vi "CTRE_Phoenix_MotorControl_ConfigReverseLimitSwitch_Enhanced.vi"(0 "CTRE Motor Controller Device Ref":T3={"DeviceStatus"={"status"=FALSE, "code"=0, "source"=""}, "Type"=enum."PWM", "PWM"={"PWM Channel"=enum."PWM 1", "DeadBand"={"Name"="", "maxPositivePwm"=0, "minPositivePwm"=0, "centerPwm"=0, "maxNegativePwm"=0, "minNegativePwm"=0, "angularRange"=0}}, "CAN"={"Device Number"=0, "SetOutput VI Ref"=variant(enum8{"Percent VBus", "Current", "Speed", "Position", "Voltage"} enum."Percent VBus"), "GetOutput VI Ref"=variant(refnum<k1> refnum), "Enable VI Ref"=variant(dbl 12.0), "Disable VI Ref"=variant(enum8{"Percent VBus", "Speed", "Position", "Slave", "Unchanged / Invalid", "Voltage Compensation", "Current", "Motion Profile"} enum."Percent VBus"), "Data"=variant}, "Invert"=FALSE}, 5 "Limit Switch Source":T2, 7 "NormallyOpenOrClosed":T1, 9 "deviceID":i32, 11 "error in (no error)":errorcluster) -> (4 "CTRE Motor Controller Device Ref":T3={"DeviceStatus"={"status"=FALSE, "code"=0, "source"=""}, "Type"=enum."PWM", "PWM"={"PWM Channel"=enum."PWM 1", "DeadBand"={"Name"="", "maxPositivePwm"=0, "minPositivePwm"=0, "centerPwm"=0, "maxNegativePwm"=0, "minNegativePwm"=0, "angularRange"=0}}, "CAN"={"Device Number"=0, "SetOutput VI Ref"=variant(enum8{"Percent VBus", "Current", "Speed", "Position", "Voltage"} enum."Percent VBus"), "GetOutput VI Ref"=variant(refnum<k1> refnum), "Enable VI Ref"=variant(dbl 12.0), "Disable VI Ref"=variant(enum8{"Percent VBus", "Speed", "Position", "Slave", "Unchanged / Invalid", "Voltage Compensation", "Current", "Motion Profile"} enum."Percent VBus"), "Data"=variant}, "Invert"=FALSE}, 15 "error out":errorcluster)   [LabVIEW 2016]
doc: "Configures the reverse limit switch.\n\n<B>Limit Switch Source</B> indicates the source of the limit switch, whether local (feedback connector) or from a remote device.\n\n<B>deviceID</B> must be set if using a remote limit switch."
uses:
  <vilib>/Rock Robotics/WPI/MotorControl/WPI_MotorControlDeviceRef.ctl
  <vilib>/Rock Robotics/WPI/MotorControl/WPI_MotorControlType.ctl
  <vilib>/Rock Robotics/SystemInterfaces/DIO/FPGA_DIOPWMChannel.ctl
  <vilib>/Rock Robotics/WPI/PWM/WPI_PWMDeadband.ctl
  Controls/CTRE_Phoenix_MotorControl_LimitSwitchSource_Local.ctl
  Controls/CTRE_Phoenix_MotorControl_LimitSwitchNormal.ctl
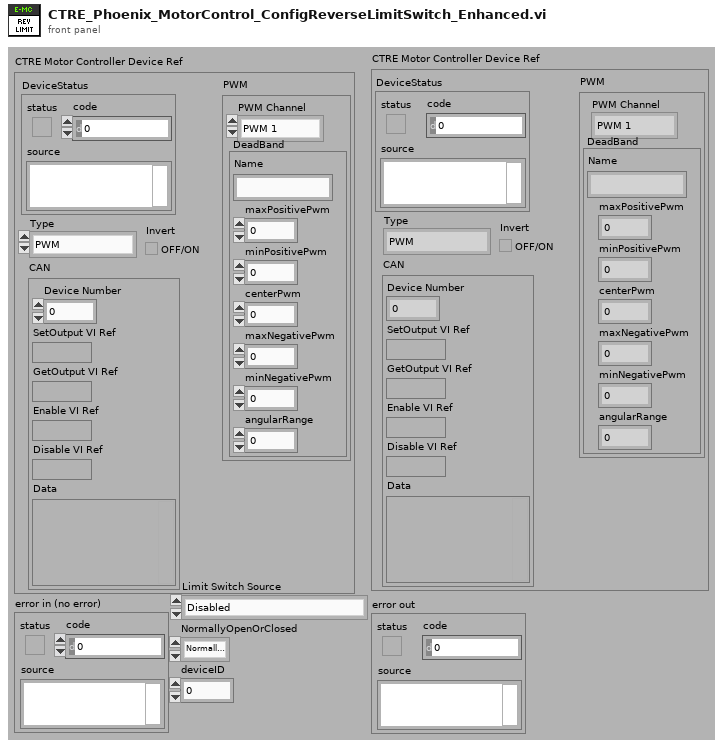
[diagram p1: front panel]
types:
  T1 = typedef "CTRE_Phoenix_MotorControl_LimitSwitchNormal.ctl" = enum16{"Normally Open", "Normally Closed"}
  T2 = typedef "CTRE_Phoenix_MotorControl_LimitSwitchSource_Local.ctl" = enum16{"Disabled", "FeedbackConnector", "RemoteTalonSRX", "RemoteCANifier"}
  T3 = typedef "WPI_MotorControlDeviceRef.ctl" = cluster{"DeviceStatus":errorcluster, "Type":T4, "PWM":cluster{"PWM Channel":T5, "DeadBand":T6}, "CAN":cluster{"Device Number":u8, "SetOutput VI Ref":variant, "GetOutput VI Ref":variant, "Enable VI Ref":variant, "Disable VI Ref":variant, "Data":variant}, "Invert":bool}
  T4 = typedef "WPI_MotorControlType.ctl" = enum16{"PWM", "CAN"}
  T5 = typedef "FPGA_DIOPWMChannel.ctl" = enum8{"PWM 0", "PWM 1", "PWM 2", "PWM 3", "PWM 4", "PWM 5", "PWM 6", "PWM 7", "PWM 8", "PWM 9", "PWM MXP 0", "PWM MXP 1", "PWM MXP 2", "PWM MXP 3", "PWM MXP 4", "PWM MXP 5", "PWM MXP 6", "PWM MXP 7", "PWM MXP 8", "PWM MXP 9", "Invalid"}
  T6 = typedef "WPI_PWMDeadband.ctl" = cluster{"Name":string, "maxPositivePwm":i32, "minPositivePwm":i32, "centerPwm":i32, "maxNegativePwm":i32, "minNegativePwm":i32, "angularRange":u16}
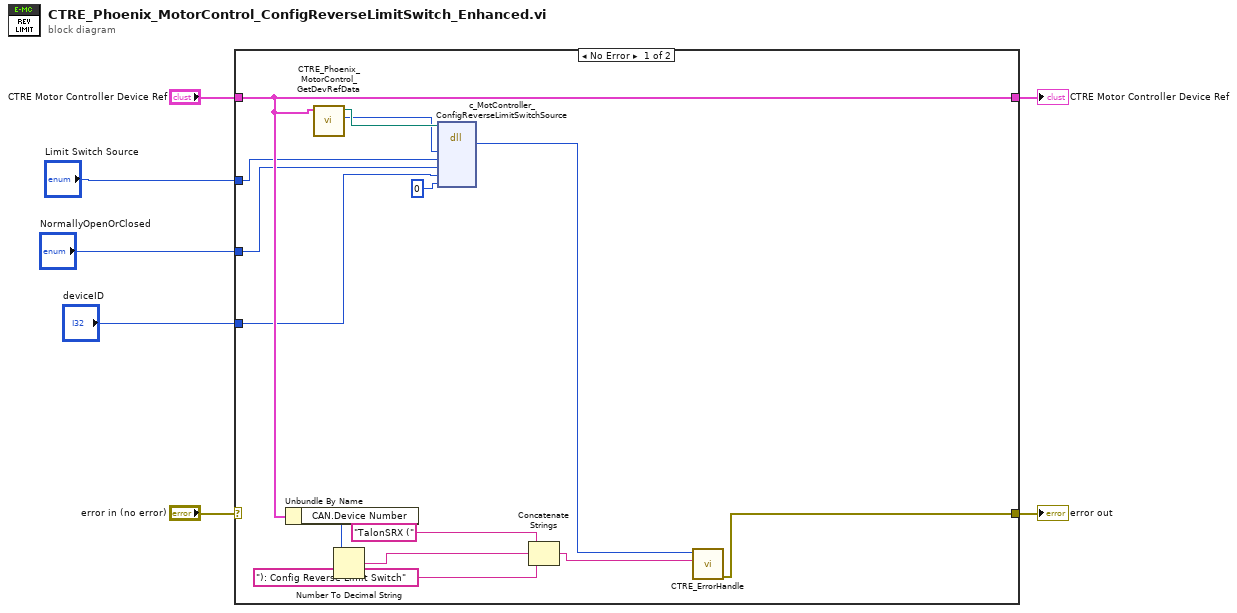
[diagram p0: block diagram]
diagram:
  n1 = case shown="No Error" "error in (no error)" {
    selector: "error in (no error)" -> [_ w23]
    tunnel: [w14 w23] -> w7
    tunnel: "CTRE Motor Controller Device Ref" -> [w17 w22]
    tunnel: [w17 w22] -> w5
    tunnel: "Limit Switch Source" -> [w10 _]
    tunnel: "NormallyOpenOrClosed" -> [w9 _]
    tunnel: "deviceID" -> [w8 _]
    frame No Error {
      n2 = Unbundle By Name(w17) -> ("CAN.Device Number"=w18:u8)
      n3 = call "CTRE_Phoenix_MotorControl_GetDevRefData.vi"("MotorControlDevRef"=w17) -> ("handle"=w11:u64, "Library"=w12:path)  [unwired: 4 in, 5 out]
      n4 = Number To Decimal String(number=w18) -> (decimal integer string=w20:string)  [unwired: 1 in]
      n5 = dll-call lib="?" fn="c_MotController_ConfigReverseLimitSwitchSource"(path in=w12, "handle"=w11, "type"=w10, "normalOpenOrClose"=w9, "deviceID"=w8, "timeoutMs"=u32 0) -> ("ErrorCode"=w15:i32)  [unwired: 7 in, 2 out]
      n6 = Concatenate Strings("TalonSRX (" ("string"), w20, "): Config Reverse Limit Switch" ("string")) -> (w13:string)
      n7 = call "CTRE_ErrorHandle.vi"("origin"=w13, "code"=w15) -> ("error out"=w14:errorcluster)  [unwired: 9 in]
    }
    frame Error {
    }
  }
  "CTRE Motor Controller Device Ref" <- w5
  "error out" <- w7
